vi "PowerMeter.vi"(3 "Error In":errorcluster, 4 "Set Wavelength (nm)":dbl=457.0, 5 "VISA resource name":refnum<visa-resource-name>="USB0::0x1313::0x807B::190927109::0::INSTR") -> (0 "Error Out":errorcluster, 1 "Power Value":dbl caption="Optical Power [W]" format="%0#3_3p", 2 "instrument handle out":refnum<visa-resource-name>)   [LabVIEW 2019]
panel:
  in  "Status":bool
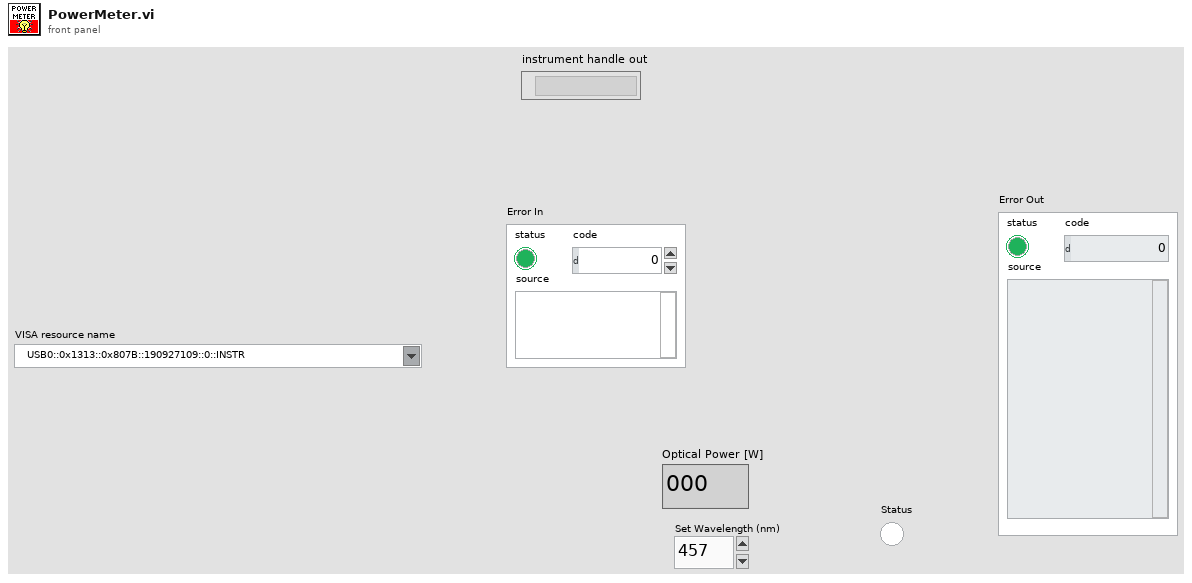
[diagram p1: front panel]
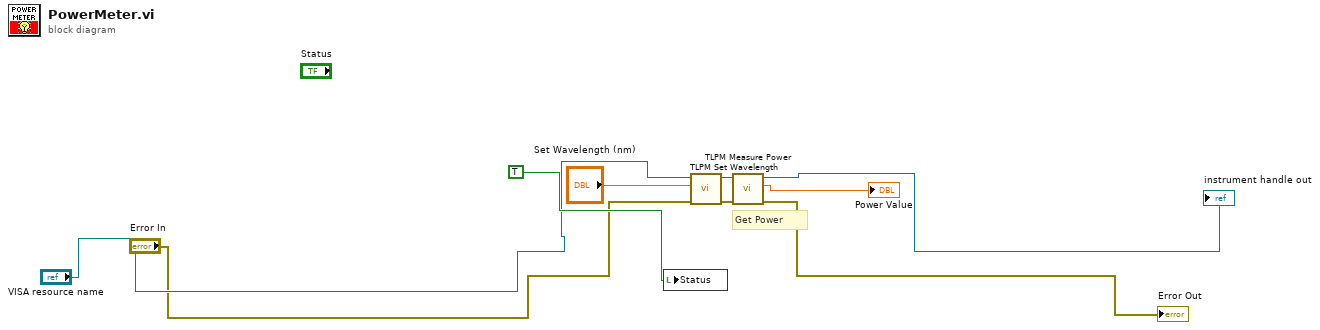
[diagram p0: block diagram]
diagram:
  # "Get Power"
  n1 = local write "Status"(TRUE ("Active")) -> ()
  n2 = call <instrlib>:"TLPM Set Wavelength.vi"("error in (no error)"="Error In", "Wavelength (0.0)"="Set Wavelength (nm)", "instrument handle"="VISA resource name") -> ("error out"=w3:errorcluster, "instrument handle out"=w4:refnum<visa-resource-name>)  [unwired: 7 in]
  n3 = call <instrlib>:"TLPM Measure Power.vi"("error in (no error)"=w3, "instrument handle"=w4) -> ("error out"=→"Error Out":errorcluster, "Power"=→"Power Value":dbl, "instrument handle out"=→"instrument handle out":refnum<visa-resource-name>)  [unwired: 7 in]
